vi "DETRead-Com-Exec.vi"(6 "All":bool, 7 "Control queue":refnum<queue>, 8 "entrée d'erreur (pas d'erreur)":errorcluster, 9 "Forever":bool=TRUE, 10 "data":variant, 11 "Detector en entrée":refnum<class "Detector.lvclass">) -> (0 "sortie d'erreur":errorcluster, 1 "#PP":i32, 2 "Spectra":cluster{"wavelengths":dbl[], "Tableau":dbl[]}[](graph), 3 "Detector out":refnum<class "Detector.lvclass">)   [LabVIEW 2015, in "Detector.lvclass"]
uses:
  Detector.lvclass
  dependecies/ControlsVIs/Clusters-def/Det-Read.ctl
  dependecies/ControlsVIs/Clusters-def/Parameters_measurement_def.ctl
  dependecies/ControlsVIs/Clusters-def/Message types.ctl
  Detector.lvclass/Detector.ctl
  Message/Message.lvclass
  GeneralFunctionality/GeneralFunctionality.lvclass
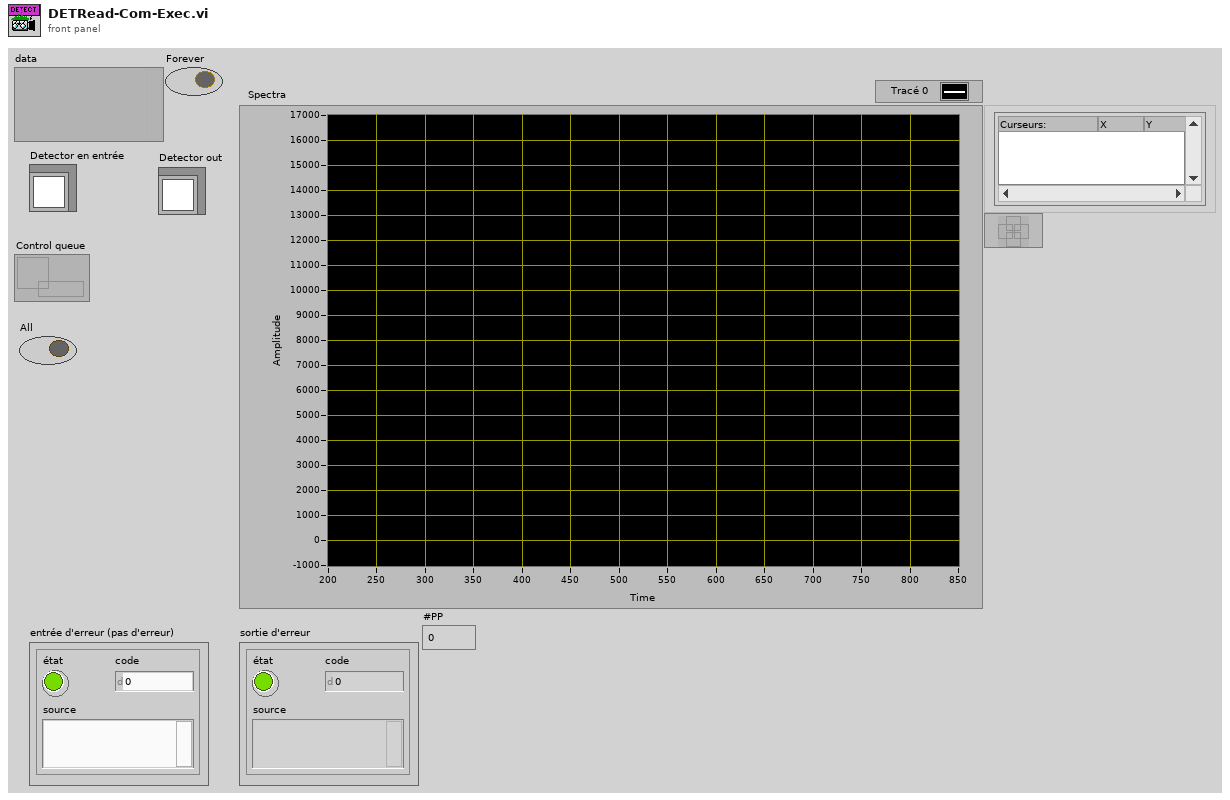
[diagram p1: front panel]
types:
  T1 = typedef "Detector.lvclass/Det-Read.ctl" = cluster{"# scans":i32, "All":bool, "Parameters of measurement":T2}
  T2 = typedef "Parameters_measurement_def.ctl" = cluster{"ODmin":dbl, "ODmax":dbl, "Aq contol":enum32{"fixed", "automatic", "fixed-auto"}, "Wavelength_fix_index":i32, "WCM_limits":cluster{"WCM_min":dbl, "WCM_max":dbl, "WCM_value":dbl}, "WCM_corrections":bool, "#cycles max":i32}
  T3 = typedef "Message types.ctl" = string
  T4 = typedef "Detector.lvclass/Def_signals_from_DET.ctl" = cluster{"xscale":sgl[], "TRABS":sgl[], "BGI":i32[][], "BGII":i32[][], "IeI":i32[][], "IeII":i32[][], "I0I":i32[][], "I0II":i32[][], "mean WCM corr cof":dbl}
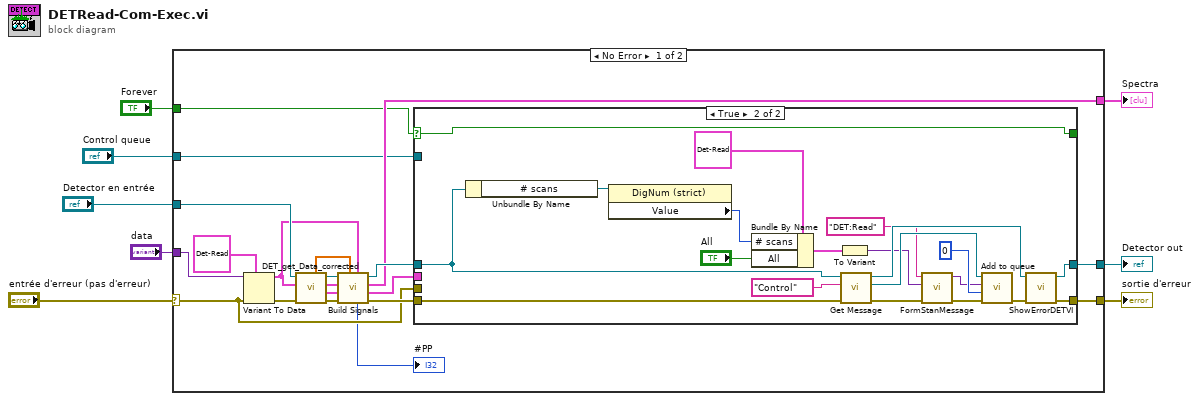
[diagram p0: block diagram]
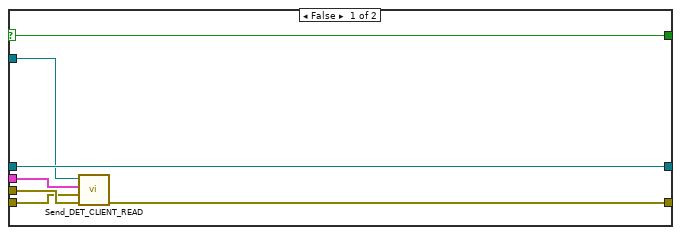
[diagram p2: hidden frame]
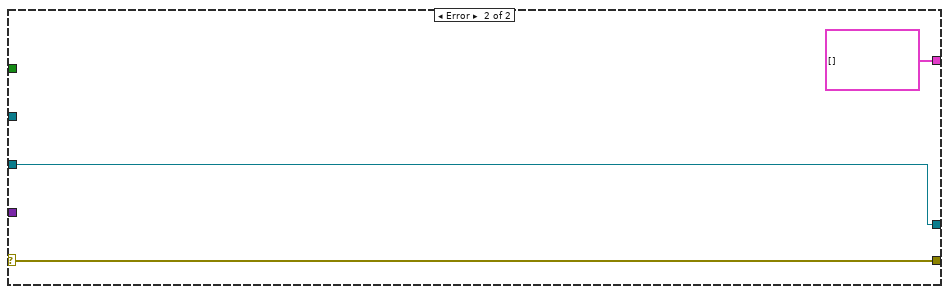
[diagram p3: hidden frame]
diagram:
  n1 = case shown="No Error" "entrée d'erreur (pas d'erreur)" {
    selector: "entrée d'erreur (pas d'erreur)" -> [w11 w57]
    tunnel: [w24 w57] -> w8
    tunnel: "Detector en entrée" -> [w14 w58]
    tunnel: [w23 w58] -> w6
    tunnel: "data" -> [w13 _]
    tunnel: [w22 cluster{"wavelengths":dbl[], "Tableau":dbl[]}[] [] ("Signals")] -> w3
    tunnel: "Forever" -> [w21 _]
    tunnel: "Control queue" -> [w20 _]
    frame No Error {
      n2 = Variant To Data(error in=w11, type=T1 {"# scans"=0, "All"=FALSE, "Parameters of measurement"={"ODmin"=0.0, "ODmax"=0.0, "Aq contol"=enum."fixed", "Wavelength_fix_index"=640, "WCM_limits"={"WCM_min"=0.0, "WCM_max"=0.0, "WCM_value"=0.0}, "WCM_corrections"=FALSE, "#cycles max"=5}} ("cluster"), Variant=w13) -> (data=w9:T1, error out=w12:errorcluster)
      n3 = call "DET_get_Data_corrected.vi"("error in (no error)"=w12, "Control IN"=w9, "Detector in"=w14) -> ("error out"=w28:errorcluster, "II channel seq"=w18:cluster{"BG":i32[], "Ie":i32[], "I0":i32[]}[], "I channel seq"=w17:cluster{"BG":i32[], "Ie":i32[], "I0":i32[]}[], "Detector out"=w27:refnum<class "Detector.lvclass">, "WCM_correction_coff"=w16:sgl[])  [unwired: 4 in]
      n4 = call-dynamic "Build Signals.vi"("Controln"=w9, "WCM_values"=w16, "error in (no error)"=w28, "II channel seq"=w18, "I channel seq"=w17, "Detector in"=w27) -> ("error out"=w25:errorcluster, "Signals so Send"=w19:T4, "Signals"=w22:cluster{"wavelengths":dbl[], "Tableau":dbl[]}[], "Detector out"=w26:refnum<class "Detector.lvclass">, "#PP"=→"#PP":i32)  [unwired: 1 in]
      n5 = case shown="True" w21 {
        selector: w21 -> [w35 w55]
        tunnel: w26 -> [w34 w44]
        tunnel: w25 -> [w31 w53]
        tunnel: [w30 w48] -> w24
        tunnel: [w35 w55] -> _
        tunnel: [w34 w46] -> w23
        tunnel: w20 -> [w33 _]
        tunnel: w19 -> [w29 _]
        tunnel: w11 -> [w32 _]
        frame False {
          n6 = call "Send_DET_CLIENT_READ.vi"("error in (no error)"=w32, "error to send"=w31, "Signals so Send"=w29, "Queue in"=w33) -> ("error out"=w30:errorcluster)  [unwired: 7 in]
        }
        frame True {
          n7 = Unbundle By Name(w44) -> ("# scans"=w43:refnum<vi>)
          n8 = property class="DigNum (strict)"(reference=w43) -> ("Value"=w42:i32)  [unwired: 1 in, 2 out]
          n9 = Bundle By Name(cluster=T1 {"# scans"=0, "All"=FALSE, "Parameters of measurement"={"ODmin"=0.0, "ODmax"=0.0, "Aq contol"=enum."fixed", "Wavelength_fix_index"=640, "WCM_limits"={"WCM_min"=0.0, "WCM_max"=0.0, "WCM_value"=0.0}, "WCM_corrections"=FALSE, "#cycles max"=5}}, "# scans"=w42, "All"="All") -> (w51:T1)
          n10 = To Variant(anything=w51) -> (Variant=w40:variant)
          n11 = call "Get Message.vi"("error in (no error)"=w53, "Message type"=T3 "Control", "GeneralFunctionality en entrée"=w44) -> ("error out"=w39:errorcluster, "Message.lvclass"=w52:refnum<class "Message.lvclass">, "GeneralFunctionality en sortie"=w47:refnum<class "Detector.lvclass">)  [unwired: 6 in]
          n12 = call "FormStanMessage.vi"("error in"=w39, "data"=w40, "Command"="DET:Read" ("command")) -> ("error out"=w38:errorcluster, "message"=w37:variant)  [unwired: 7 in]
          n13 = call "Add to queue.vi"("error in (no error)"=w38, "timeout in ms (-1)"=0, "Data"=w37, "Message in"=w52) -> ("error out"=w49:errorcluster)  [unwired: 6 in, 1 out]
          n14 = call "ShowErrorDETVI.vi"("error in (no error)"=w49, "Detector in"=w47) -> ("error out"=w48:errorcluster, "Detector out"=w46:refnum<class "Detector.lvclass">)  [unwired: 8 in]
        }
      }
    }
    frame Error {
    }
  }
  "sortie d'erreur" <- w8
  "Detector out" <- w6
  "Spectra" <- w3
